vi "AlliGator Pad or Truncate Decay.vi"(8 "Error In":errorcluster, 9 "# Requested Points":i32, 11 "Plot in":cluster{"Axis":dbl[], "Histogram":dbl[]}) -> (0 "Error Out":errorcluster, 3 "Plot out":cluster{"Axis":dbl[], "Histogram":dbl[]})   [LabVIEW 2021, in "AlliGator Fit Method Benchmark.lvlib"]
doc: "Adds or removes decay points for it to match the laser period."
uses:
  AlliGator Fit Method Benchmark.lvlib
  66de7b3f-7c31-4139-912e-c4e08d862171.vi
  <vilib>/Analysis/NI_AALBase.lvlib
panel:
  # "see the AlliGator License on the block diagram (Ctrl+E or Window:Show Block Diagram)"
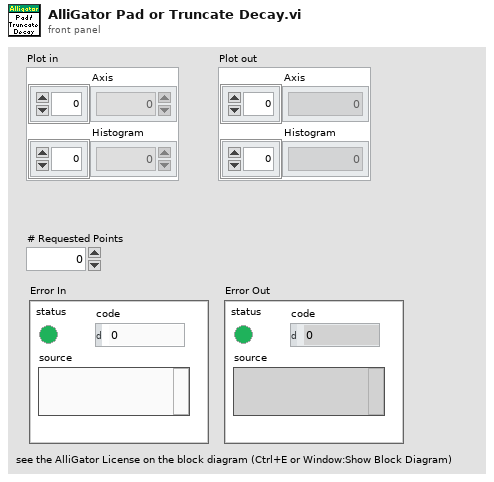
[diagram p1: front panel]
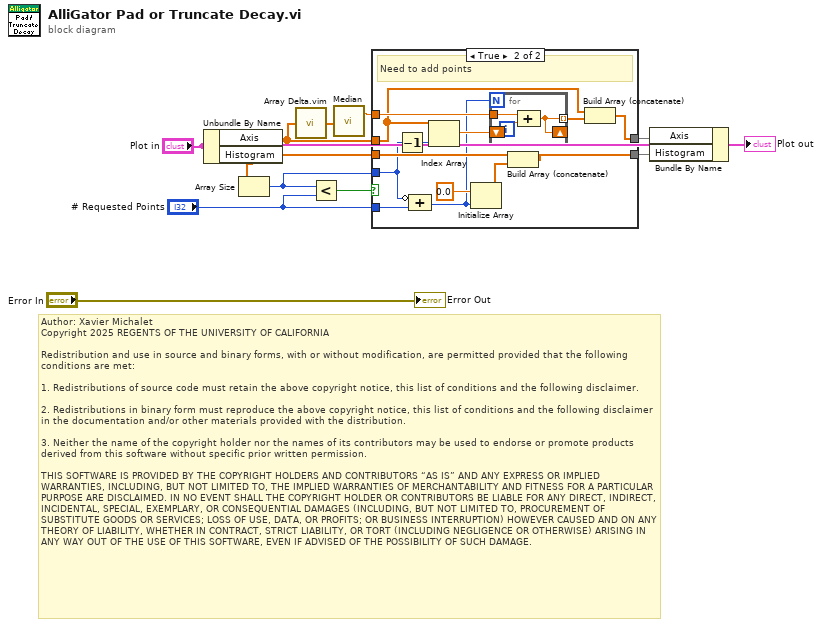
[diagram p0: block diagram]
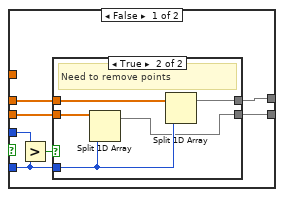
[diagram p2: hidden frame]
diagram:
  # "Author: Xavier Michalet\nCopyright 2025 REGENTS OF THE UNIVERSITY OF CALIFORNIA\n\nRedistribution and use in source and binary forms, with or without modification, are permitted provided that the following conditions are met:\n\n1. Redistributions of source code must retain the above copyright notice, this list of conditions and the following disclaimer.\n\n2. Redistributions in binary form must reproduce the above copyright notice, this list of conditions and the following disclaimer in the documentation and/or other materials provided with the distribution.\n\n3. Neither the name of the copyright holder nor the names of its contributors may be used to endorse or promote products derived from this software without specific prior written permission.\n\nTHIS SOFTWARE IS PROVIDED BY THE COPYRIGHT HOLDERS AND CONTRIBUTORS “AS IS” AND ANY EXPRESS OR IMPLIED WARRANTIES, INCLUDING, BUT NOT LIMITED TO, THE IMPLIED WARRANTIES OF MERCHANTABILITY AND FITNESS FOR A PARTICULAR PURPOSE ARE DISCLAIMED. IN NO EVENT SHALL THE COPYRIGHT HOLDER OR CONTRIBUTORS BE LIABLE FOR ANY DIRECT, INDIRECT, INCIDENTAL, SPECIAL, EXEMPLARY, OR CONSEQUENTIAL DAMAGES (INCLUDING, BUT NOT LIMITED TO, PROCUREMENT OF SUBSTITUTE GOODS OR SERVICES; LOSS OF USE, DATA, OR PROFITS; OR BUSINESS INTERRUPTION) HOWEVER CAUSED AND ON ANY THEORY OF LIABILITY, WHETHER IN CONTRACT, STRICT LIABILITY, OR TORT (INCLUDING NEGLIGENCE OR OTHERWISE) ARISING IN ANY WAY OUT OF THE USE OF THIS SOFTWARE, EVEN IF ADVISED OF THE POSSIBILITY OF SUCH DAMAGE."
  n1 = Unbundle By Name("Plot in") -> ("Axis"=w8:dbl[], "Histogram"=w6:dbl[])
  n2 = Array Size(array=w6) -> (size(s)=w9:i32)
  n3 = call "Array Delta.vim"("A"=w8) -> ("A[i+1]-A[i]"=w7:dbl[])  [unwired: 8 in]
  n4 = Less?(x=w9, y="# Requested Points") -> (x < y?=w11:bool)
  n5 = call <vilib>:"Median.vi"("X"=w7) -> ("median"=w1:dbl)  [unwired: 1 out]
  n6 = case shown="True" w11 {
    tunnel: "# Requested Points" -> [w16 w39]
    tunnel: w9 -> [w19 w34]
    tunnel: w8 -> [w17 w29]
    tunnel: w6 -> [w14 w37]
    tunnel: [w13 w35] -> w3
    tunnel: [w15 w28] -> w5
    tunnel: w1 -> [_ w31]
    frame False {
      n7 = Greater?(x=w19, y=w16) -> (0:w18:bool)
      n8 = case shown="True" w18 {
        tunnel: w17 -> [w21 w26]
        tunnel: w16 -> [_ w23]
        tunnel: [w21 w25] -> w15
        tunnel: w14 -> [w20 w24]
        tunnel: [w20 w22] -> w13
        frame False {
        }
        frame True {
          # "Need to remove points"
          n9 = Split 1D Array(array=w24, index=w23) -> (first subarray=w22:dbl[])  [unwired: 1 out]
          n10 = Split 1D Array(array=w26, index=w23) -> (first subarray=w25:dbl[])  [unwired: 1 out]
        }
      }
    }
    frame True {
      # "Need to add points"
      n11 = Decrement(x=w34) -> (x-1=w33:i32)
      n12 = Compound Arithmetic op=ADD(invert w34, w39) -> (w27:i32)
      n13 = Index Array(array=w29, index=w33) -> (element=w32:dbl)
      n14 = Initialize Array(0.0 ("element"), w27) -> (w36:dbl[])
      n15 = for {
        N: w27 -> [_]
        shift-right: [w40] -> _
        shift-left: w32 -> [w42]
        tunnel: w31 -> [w41]
        tunnel: [w40] -> w30 mode=indexing
        n16 = Compound Arithmetic op=ADD(w41, w42) -> (w40:dbl)
      }
      n17 = Build Array (concatenate)(w37, w36) -> (w35:dbl[])
      n18 = Build Array (concatenate)(w29, w30) -> (w28:dbl[])
    }
  }
  n19 = Bundle By Name(cluster="Plot in", "Axis"=w5, "Histogram"=w3) -> (→"Plot out":cluster{"Axis":dbl[], "Histogram":dbl[]})
  "Error Out" <- "Error In"
